vi "SetChanSel.vi"(8 "错误输入（无错误）":errorcluster, 10 "ChanSel":bool[](array[boolean])=[TRUE, TRUE, TRUE, TRUE, TRUE, TRUE, TRUE, TRUE, FALSE, FALSE, FALSE, FALSE, FALSE, FALSE, FALSE, FALSE], 11 "DevIndex":i32) -> (0 "错误输出":errorcluster, 2 "ChanSel":u16, 3 "DevIndex Output":i32)   [LabVIEW 2018]
panel:
  out "ErroCode":i32
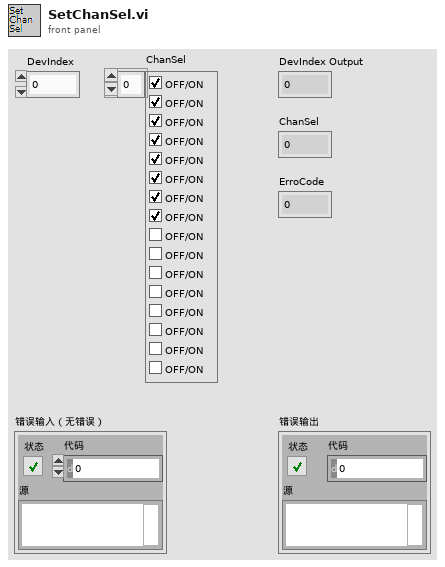
[diagram p1: front panel]
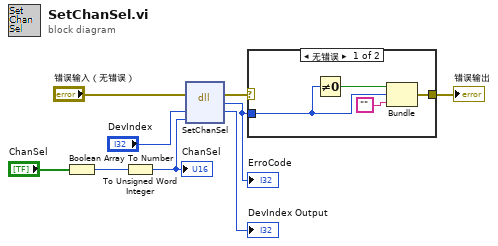
[diagram p0: block diagram]
diagram:
  n1 = Boolean Array To Number(Boolean array="ChanSel") -> (number=w6:u32)
  n2 = To Unsigned Word Integer(number=w6) -> (unsigned 16bit integer=w4:u16)
  "ChanSel" <- w4
  n3 = dll-call lib="PTH2@abs H科研项目仅一项目程序32位usb-1000.dll" fn="SetChanSel"(error in="错误输入（无错误）", "DevIndex"="DevIndex", "ChanSel"=w4) -> (error out=w3:errorcluster, "ErroCode"=w2:i32, "DevIndex"=→"DevIndex Output":i32)  [unwired: 3 in, 1 out]
  "ErroCode" <- w2
  n4 = case shown="无错误" w3 {
    selector: w3 -> [_ w14]
    tunnel: [w11 w14] -> w1
    tunnel: w2 -> [w12 _]
    frame No Error {
      n5 = Not Equal To 0?(x=w12) -> (x != 0?=w13:bool)
      n6 = Bundle(w13, "ErroCode"=w12, "") -> (w11:cluster{bool, "ErroCode":i32, string})  [unwired: 1 in]
    }
    frame Error {
    }
  }
  "错误输出" <- w1
